vi "Add Device.vi"(8 "error in (no error)":errorcluster, 11 "picoG in":refnum<class "picoG.lvclass">) -> (0 "error out":errorcluster, 3 "picoG out":refnum<class "picoG.lvclass">)   [LabVIEW 2020, in "PicoG-App.lvlib" / "picoG.lvclass"]
uses:
  picoG.lvclass
  picoG.lvclass/picoG.ctl
  Builds/picoG/ppl/PicoG-Core.lvlibp/PicoG-Processor/PicoG-Core/Platform/Platform.lvclass
  Device/Device.lvclass
  Builds/picoG/ppl/PicoG-Core.lvlibp/PicoG-Processor/PicoG-Core/PlatformManager/PlatformManager.lvclass
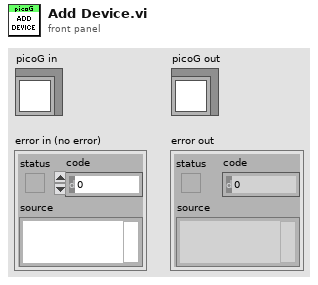
[diagram p1: front panel]
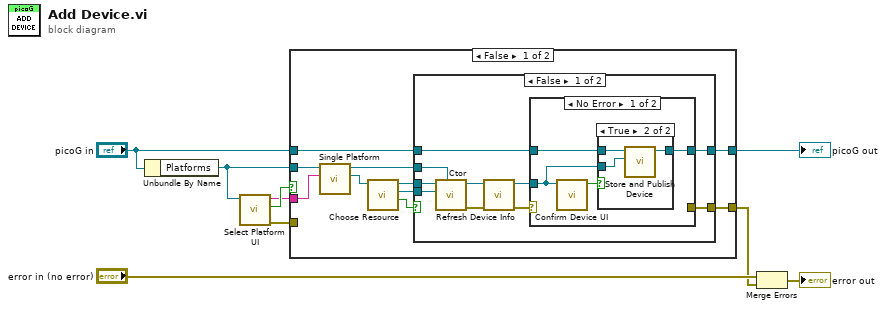
[diagram p0: block diagram]
diagram:
  n1 = Unbundle By Name("picoG in") -> ("Platforms"=w5:refnum<class "PlatformManager.lvclass">)
  n2 = call "Select Platform UI.vi"("Plugins"=w5) -> ("error out"=w7:errorcluster, "Cancelled"=w9:bool, "Platform"=w8:string)  [unwired: 8 in]
  n3 = case shown="False" w9 {
    tunnel: w8 -> [w18 _]
    tunnel: w7 -> [_ _]
    tunnel: "picoG in" -> [w15 w41]
    tunnel: w5 -> [w19 _]
    tunnel: [w14 w41] -> w4
    tunnel: [w11 _] -> w1
    frame False {
      n4 = call "Single Platform.vi"("Platform Name"=w18, "PlatformManager in"=w19) -> ("Platform"=w17:refnum<class "Platform.lvclass">, "PlatformManager out"=w10:refnum<class "PlatformManager.lvclass">)  [unwired: 7 in, 1 out]
      n5 = call-dynamic "Choose Resource.vi"("DeployTarget in"=w17) -> ("Cancelled"=w16:bool, "Resource"=w12:refnum<class "Resource.lvclass">, "DeployTarget out"=w13:refnum<class "Platform.lvclass">)  [unwired: 7 in, 1 out]
      n6 = case shown="False" w16 {
        tunnel: w15 -> [w25 w40]
        tunnel: [w24 w40] -> w14
        tunnel: w13 -> [w29 _]
        tunnel: w12 -> [w28 _]
        tunnel: [w21 _] -> w11
        tunnel: w10 -> [w20 _]
        frame False {
          n7 = call "Ctor.vi"("Platforms"=w20, "Resource"=w28, "Platform"=w29) -> ("error out"=w26:errorcluster, "Device out"=w27:refnum<class "Device.lvclass">)  [unwired: 7 in]
          n8 = call "Refresh Device Info.vi"("error in (no error)"=w26, "Device in"=w27) -> ("error out"=w22:errorcluster, "Device out"=w23:refnum<class "Device.lvclass">)  [unwired: 8 in]
          n9 = case shown="No Error" w22 {
            selector: w22 -> [_ w39]
            tunnel: w25 -> [w32 w38]
            tunnel: [w31 w38] -> w24
            tunnel: w23 -> [w30 _]
            tunnel: [_ w39] -> w21
            frame No Error {
              n10 = call "Confirm Device UI.vi"("Device"=w30) -> ("Confirmed"=w33:bool)  [unwired: 10 in]
              n11 = case shown="True" w33 {
                tunnel: w32 -> [w34 w37]
                tunnel: [w34 w36] -> w31
                tunnel: w30 -> [_ w35]
                frame False {
                }
                frame True {
                  n12 = call "Store and Publish Device.vi"("Device"=w35, "picoG in"=w37) -> ("picoG out"=w36:refnum<class "picoG.lvclass">)  [unwired: 8 in, 1 out]
                }
              }
            }
            frame Error {
            }
          }
        }
        frame True {
        }
      }
    }
    frame True {
    }
  }
  "picoG out" <- w4
  n13 = Merge Errors("error in (no error)", w1) -> (→"error out":errorcluster)
